vi "FilterEmptyStrings.vi"(8 "error in":errorcluster, 11 "Array in":string[](array[string])) -> (0 "error out":errorcluster, 3 "Array out":string[](array[string]))   [LabVIEW 2017]
doc: "Removes any empty string in the string array"
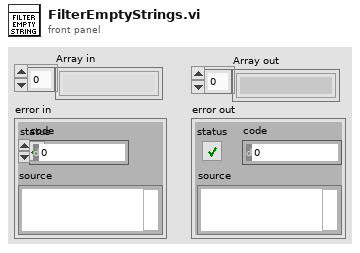
[diagram p1: front panel]
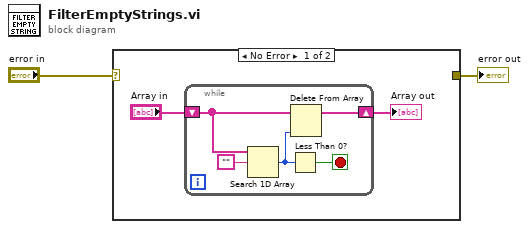
[diagram p0: block diagram]
diagram:
  n1 = case shown="No Error" "error in" {
    selector: "error in" -> [_ w10]
    tunnel: [_ w10] -> w1
    frame No Error {
      n2 = while {
        shift-right: [w7] -> w4
        shift-left: "Array in" -> [w8]
        stop <- w5 stop-if-true
        n3 = Search 1D Array(1D array=w8, element="") -> (index of element=w6:i32)  [unwired: 1 in]
        n4 = Less Than 0?(x=w6) -> (x < 0?=w5:bool)
        n5 = Delete From Array(array=w8, index=w6) -> (array with subset deleted=w7:string[])  [unwired: 1 in, 1 out]
      }
      "Array out" <- w4
    }
    frame Error {
    }
  }
  "error out" <- w1
